vi "reconnect.vi"(8 "error in (no error)":errorcluster, 9 "port":u16, 10 "timeout ms (25000)":i32, 11 "WebSocket in":refnum<class "WebSocket Server.lvclass">) -> (0 "error out":errorcluster, 2 "Connected":bool, 3 "WebSocket out":refnum<class "WebSocket Server.lvclass">)   [LabVIEW 2018]
uses:
  <vilib>/MediaMongrels Ltd/WebSockets/WebSockets/WebSocket Server/WebSocket Server.lvclass
  <vilib>/MediaMongrels Ltd/WebSockets/Sockets/VISA TCP Listener/VISA TCP Listener.lvclass
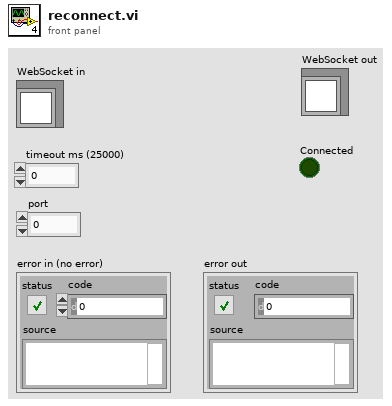
[diagram p1: front panel]
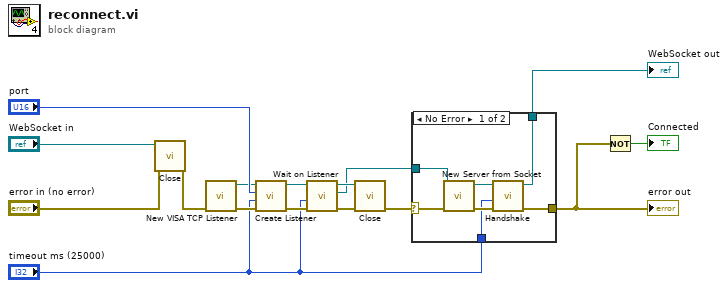
[diagram p0: block diagram]
diagram:
  n1 = call-dynamic "Close.vi"("error in (no error)"="error in (no error)", "WebSocket in"="WebSocket in") -> ("error out"=w15:errorcluster)  [unwired: 9 in]
  n2 = call <vilib>:"New VISA TCP Listener.vi"("error in (no error)"=w15) -> ("error out"=w11:errorcluster, "VISA TCP Listener out"=w12:refnum<class "VISA TCP Listener.lvclass">)  [unwired: 9 in]
  n3 = call-dynamic "Create Listener.vi"("error in (no error)"=w11, "timeout ms (5000)"="timeout ms (25000)", "Port"="port", "VISA TCP Listener in"=w12) -> ("error out"=w9:errorcluster, "VISA TCP Listener out"=w7:refnum<class "VISA TCP Listener.lvclass">)  [unwired: 6 in]
  n4 = call-dynamic "Wait on Listener.vi"("error in (no error)"=w9, "timeout ms (5000)"="timeout ms (25000)", "VISA TCP Listener in"=w7) -> ("error out"=w10:errorcluster, "Socket out"=w6:refnum<class "Socket.lvclass">, "VISA TCP Listener out"=w8:refnum<class "VISA TCP Listener.lvclass">)  [unwired: 6 in]
  n5 = call-dynamic "Close.vi"("error in (no error)"=w10, "VISA TCP Listener in"=w8) -> ("error out"=w1:errorcluster)  [unwired: 9 in]
  n6 = case shown="No Error" w1 {
    selector: w1 -> [w17 w24]
    tunnel: w6 -> [w21 _]
    tunnel: [w20 _] -> w5
    tunnel: "timeout ms (25000)" -> [w19 _]
    tunnel: [w18 w24] -> w3
    frame No Error {
      n7 = call <vilib>:"New Server from Socket.vi"("error in (no error)"=w17, "Socket"=w21) -> ("error out"=w22:errorcluster, "WebSocket Server out"=w23:refnum<class "WebSocket Server.lvclass">)  [unwired: 8 in]
      n8 = call-dynamic "Handshake.vi"("error in (no error)"=w22, "timeout ms (5000)"=w19, "WebSocket Connection in"=w23) -> ("error out"=w18:errorcluster, "WebSocket Connection out"=w20:refnum<class "WebSocket Server.lvclass">)  [unwired: 7 in]
    }
    frame Error {
    }
  }
  "WebSocket out" <- w5
  "error out" <- w3
  n9 = Not(x=w3) -> (.not. x?=→"Connected":bool)
